vi "AlliGator Compute Multiple Average Phasors (Selected Plots).vi"(8 "error in (no error)":errorcluster, 9 "Phasor Frequency":dbl[unit]=160000000.0 format="%#_4g", 10 "Lifetime Graph Ref":refnum<vi>, 11 "Phasor Graph Ref":refnum<vi>) -> (0 "error out":errorcluster, 1 "Phasor SDV Plot":cluster{"Array":dbl[], "Array":dbl[]}, 2 "Average Phasor Plot":cluster{"Array":dbl[], "Array":dbl[]}, 4 "Result String":string)   [LabVIEW 2021, in "AlliGator Phasor Graph.lvlib"]
doc: "Computes one average phasor (and derived quantities) per phasor plot in the Phasor Graph and plots each quantity as a series (where the abscissa is the plot index)."
uses:
  AlliGator Phasor Graph.lvlib
  Phasor/Phasor (g, s).ctl
  71c37bd2-47c7-4488-96cd-0a664e0032d0.vi/bdeb4727-ff4d-4ac9-8e28-741831c2f97b.vi
  71c37bd2-47c7-4488-96cd-0a664e0032d0.vi/144b8a7a-6b33-495e-8c76-f9961f20cf57.vi
  71c37bd2-47c7-4488-96cd-0a664e0032d0.vi/b7572d45-ec39-4925-b449-50494e6a70fe.vi
  71c37bd2-47c7-4488-96cd-0a664e0032d0.vi/1eb0ddea-bb1c-44e5-a105-a57d15a7e766.vi
  71c37bd2-47c7-4488-96cd-0a664e0032d0.vi/c6722fb2-ba6a-4669-88ce-b6a529e82caa.vi
  71c37bd2-47c7-4488-96cd-0a664e0032d0.vi/9c66b583-3c03-4ab0-9ee8-bb1b5672edcc.vi
  71c37bd2-47c7-4488-96cd-0a664e0032d0.vi/fa4085e0-ed61-4e8f-9831-aca6a4188fed.vi
  71c37bd2-47c7-4488-96cd-0a664e0032d0.vi/0c4d34e2-59e2-4c6b-a2f9-6f475d8bea3b.vi
  71c37bd2-47c7-4488-96cd-0a664e0032d0.vi/9179bf7b-4f23-4b71-844f-7bfb33db4ee4.vi
  af37836b-9043-4320-9d11-d8691fee8c1a.vi/bdeb4727-ff4d-4ac9-8e28-741831c2f97b.vi
  af37836b-9043-4320-9d11-d8691fee8c1a.vi/144b8a7a-6b33-495e-8c76-f9961f20cf57.vi
  af37836b-9043-4320-9d11-d8691fee8c1a.vi/b7572d45-ec39-4925-b449-50494e6a70fe.vi
  af37836b-9043-4320-9d11-d8691fee8c1a.vi/1eb0ddea-bb1c-44e5-a105-a57d15a7e766.vi
  af37836b-9043-4320-9d11-d8691fee8c1a.vi/c6722fb2-ba6a-4669-88ce-b6a529e82caa.vi
  af37836b-9043-4320-9d11-d8691fee8c1a.vi/9c66b583-3c03-4ab0-9ee8-bb1b5672edcc.vi
  af37836b-9043-4320-9d11-d8691fee8c1a.vi/fa4085e0-ed61-4e8f-9831-aca6a4188fed.vi
  af37836b-9043-4320-9d11-d8691fee8c1a.vi/0c4d34e2-59e2-4c6b-a2f9-6f475d8bea3b.vi
  af37836b-9043-4320-9d11-d8691fee8c1a.vi/9179bf7b-4f23-4b71-844f-7bfb33db4ee4.vi
  bb80a456-60a4-403d-849e-61bda53aa3b6.vi/bdeb4727-ff4d-4ac9-8e28-741831c2f97b.vi
  bb80a456-60a4-403d-849e-61bda53aa3b6.vi/144b8a7a-6b33-495e-8c76-f9961f20cf57.vi
  bb80a456-60a4-403d-849e-61bda53aa3b6.vi/b7572d45-ec39-4925-b449-50494e6a70fe.vi
  bb80a456-60a4-403d-849e-61bda53aa3b6.vi/1eb0ddea-bb1c-44e5-a105-a57d15a7e766.vi
  bb80a456-60a4-403d-849e-61bda53aa3b6.vi/c6722fb2-ba6a-4669-88ce-b6a529e82caa.vi
  bb80a456-60a4-403d-849e-61bda53aa3b6.vi/9c66b583-3c03-4ab0-9ee8-bb1b5672edcc.vi
  bb80a456-60a4-403d-849e-61bda53aa3b6.vi/fa4085e0-ed61-4e8f-9831-aca6a4188fed.vi
  bb80a456-60a4-403d-849e-61bda53aa3b6.vi/0c4d34e2-59e2-4c6b-a2f9-6f475d8bea3b.vi
  bb80a456-60a4-403d-849e-61bda53aa3b6.vi/9179bf7b-4f23-4b71-844f-7bfb33db4ee4.vi
  4a9871b1-e52c-439f-b7fd-fdf7bfeb4803.vi/bdeb4727-ff4d-4ac9-8e28-741831c2f97b.vi
  4a9871b1-e52c-439f-b7fd-fdf7bfeb4803.vi/144b8a7a-6b33-495e-8c76-f9961f20cf57.vi
  4a9871b1-e52c-439f-b7fd-fdf7bfeb4803.vi/b7572d45-ec39-4925-b449-50494e6a70fe.vi
  4a9871b1-e52c-439f-b7fd-fdf7bfeb4803.vi/1eb0ddea-bb1c-44e5-a105-a57d15a7e766.vi
  4a9871b1-e52c-439f-b7fd-fdf7bfeb4803.vi/c6722fb2-ba6a-4669-88ce-b6a529e82caa.vi
  4a9871b1-e52c-439f-b7fd-fdf7bfeb4803.vi/9c66b583-3c03-4ab0-9ee8-bb1b5672edcc.vi
  4a9871b1-e52c-439f-b7fd-fdf7bfeb4803.vi/fa4085e0-ed61-4e8f-9831-aca6a4188fed.vi
  4a9871b1-e52c-439f-b7fd-fdf7bfeb4803.vi/0c4d34e2-59e2-4c6b-a2f9-6f475d8bea3b.vi
  4a9871b1-e52c-439f-b7fd-fdf7bfeb4803.vi/9179bf7b-4f23-4b71-844f-7bfb33db4ee4.vi
  ea11824e-7dc4-44cf-8e7c-2ee366fc47de.vi/bdeb4727-ff4d-4ac9-8e28-741831c2f97b.vi
  ea11824e-7dc4-44cf-8e7c-2ee366fc47de.vi/144b8a7a-6b33-495e-8c76-f9961f20cf57.vi
  ea11824e-7dc4-44cf-8e7c-2ee366fc47de.vi/b7572d45-ec39-4925-b449-50494e6a70fe.vi
  ea11824e-7dc4-44cf-8e7c-2ee366fc47de.vi/1eb0ddea-bb1c-44e5-a105-a57d15a7e766.vi
  ea11824e-7dc4-44cf-8e7c-2ee366fc47de.vi/c6722fb2-ba6a-4669-88ce-b6a529e82caa.vi
  ea11824e-7dc4-44cf-8e7c-2ee366fc47de.vi/9c66b583-3c03-4ab0-9ee8-bb1b5672edcc.vi
  ea11824e-7dc4-44cf-8e7c-2ee366fc47de.vi/fa4085e0-ed61-4e8f-9831-aca6a4188fed.vi
  ea11824e-7dc4-44cf-8e7c-2ee366fc47de.vi/0c4d34e2-59e2-4c6b-a2f9-6f475d8bea3b.vi
  ea11824e-7dc4-44cf-8e7c-2ee366fc47de.vi/9179bf7b-4f23-4b71-844f-7bfb33db4ee4.vi
  6682c489-6466-43b2-8f2f-8d331e8ea9c3.vi/bdeb4727-ff4d-4ac9-8e28-741831c2f97b.vi
  6682c489-6466-43b2-8f2f-8d331e8ea9c3.vi/144b8a7a-6b33-495e-8c76-f9961f20cf57.vi
  6682c489-6466-43b2-8f2f-8d331e8ea9c3.vi/b7572d45-ec39-4925-b449-50494e6a70fe.vi
  6682c489-6466-43b2-8f2f-8d331e8ea9c3.vi/1eb0ddea-bb1c-44e5-a105-a57d15a7e766.vi
  6682c489-6466-43b2-8f2f-8d331e8ea9c3.vi/c6722fb2-ba6a-4669-88ce-b6a529e82caa.vi
  6682c489-6466-43b2-8f2f-8d331e8ea9c3.vi/9c66b583-3c03-4ab0-9ee8-bb1b5672edcc.vi
  6682c489-6466-43b2-8f2f-8d331e8ea9c3.vi/fa4085e0-ed61-4e8f-9831-aca6a4188fed.vi
  6682c489-6466-43b2-8f2f-8d331e8ea9c3.vi/0c4d34e2-59e2-4c6b-a2f9-6f475d8bea3b.vi
  6682c489-6466-43b2-8f2f-8d331e8ea9c3.vi/9179bf7b-4f23-4b71-844f-7bfb33db4ee4.vi
  4c569add-43d7-45f2-8521-633ddc3d646c.vi/bdeb4727-ff4d-4ac9-8e28-741831c2f97b.vi
  4c569add-43d7-45f2-8521-633ddc3d646c.vi/144b8a7a-6b33-495e-8c76-f9961f20cf57.vi
  4c569add-43d7-45f2-8521-633ddc3d646c.vi/b7572d45-ec39-4925-b449-50494e6a70fe.vi
  4c569add-43d7-45f2-8521-633ddc3d646c.vi/1eb0ddea-bb1c-44e5-a105-a57d15a7e766.vi
  4c569add-43d7-45f2-8521-633ddc3d646c.vi/c6722fb2-ba6a-4669-88ce-b6a529e82caa.vi
  4c569add-43d7-45f2-8521-633ddc3d646c.vi/9c66b583-3c03-4ab0-9ee8-bb1b5672edcc.vi
  4c569add-43d7-45f2-8521-633ddc3d646c.vi/fa4085e0-ed61-4e8f-9831-aca6a4188fed.vi
  4c569add-43d7-45f2-8521-633ddc3d646c.vi/0c4d34e2-59e2-4c6b-a2f9-6f475d8bea3b.vi
  4c569add-43d7-45f2-8521-633ddc3d646c.vi/9179bf7b-4f23-4b71-844f-7bfb33db4ee4.vi
  2777646a-574b-4d4e-97c5-dbf227eafc7c.vi/bdeb4727-ff4d-4ac9-8e28-741831c2f97b.vi
  2777646a-574b-4d4e-97c5-dbf227eafc7c.vi/144b8a7a-6b33-495e-8c76-f9961f20cf57.vi
  2777646a-574b-4d4e-97c5-dbf227eafc7c.vi/b7572d45-ec39-4925-b449-50494e6a70fe.vi
  2777646a-574b-4d4e-97c5-dbf227eafc7c.vi/1eb0ddea-bb1c-44e5-a105-a57d15a7e766.vi
  2777646a-574b-4d4e-97c5-dbf227eafc7c.vi/c6722fb2-ba6a-4669-88ce-b6a529e82caa.vi
  2777646a-574b-4d4e-97c5-dbf227eafc7c.vi/9c66b583-3c03-4ab0-9ee8-bb1b5672edcc.vi
  2777646a-574b-4d4e-97c5-dbf227eafc7c.vi/fa4085e0-ed61-4e8f-9831-aca6a4188fed.vi
  2777646a-574b-4d4e-97c5-dbf227eafc7c.vi/0c4d34e2-59e2-4c6b-a2f9-6f475d8bea3b.vi
  2777646a-574b-4d4e-97c5-dbf227eafc7c.vi/9179bf7b-4f23-4b71-844f-7bfb33db4ee4.vi
  <userlib>/_OpenG.lib/array/array.llb/Filter 1D Array with Scalar (I32)__ogtk.vi
  AlliGator Abort.vi
  Graphs/XY Graph/XY Graph Add Single Plot with Name.vi
  <vilib>/Utility/error.llb/Error Cluster From Error Code.vi
  <vilib>/ErrorRing/Error Ring.xnode
  Phasor/Phasor.lvlib
  <vilib>/Analysis/NI_AALBase.lvlib
  Arrays/Arrays.lvlib
  Graphs/XY Graph/XY Graph Add-Ons.lvlib
  AlliGator Phasor Ratio.lvlib
  <userlib>/_OpenG.lib/array/array.llb/openg_array.lvlib
  AlliGator Globals, Variables & Constants.lvlib
  Strings/Strings.lvlib
  Utilities/Utilities.lvlib
  <userlib>/_OpenG.lib/array/array.llb/Filter 1D Array (DBL)__ogtk.vi
panel:
  # "see the AlliGator License on the block diagram (Ctrl+E or Window:Show Block Diagram)"
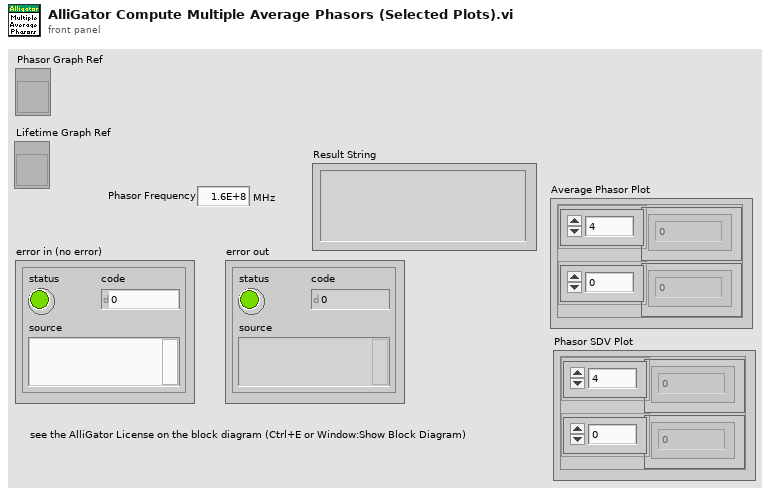
[diagram p1: front panel]
types:
  T1 = typedef "XY Graph Add-Ons.lvlib/XY Graph Refnum.ctl" = refnum<vi>
  T2 = typedef "Phasor.lvlib/Phasor (g, s).ctl" = cluster{"g":dbl, "s":dbl}
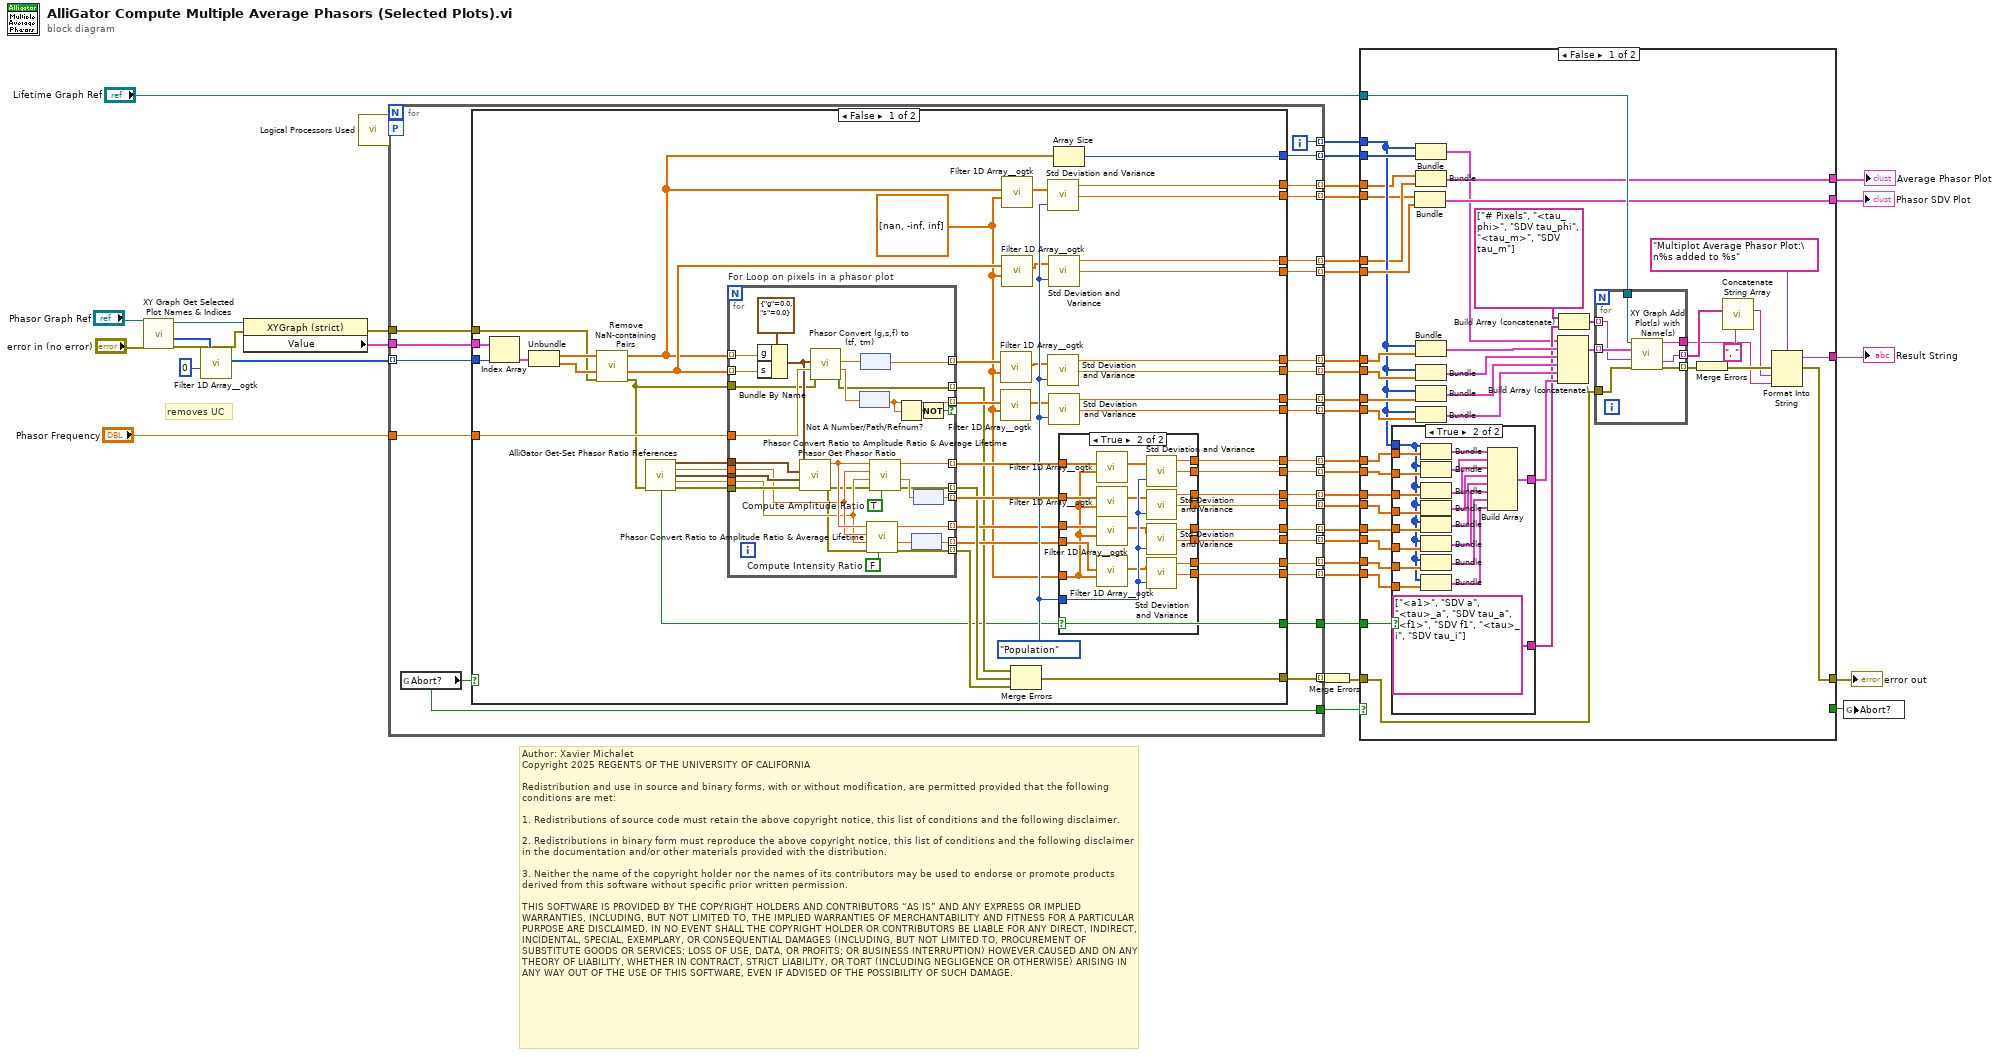
[diagram p0: block diagram]
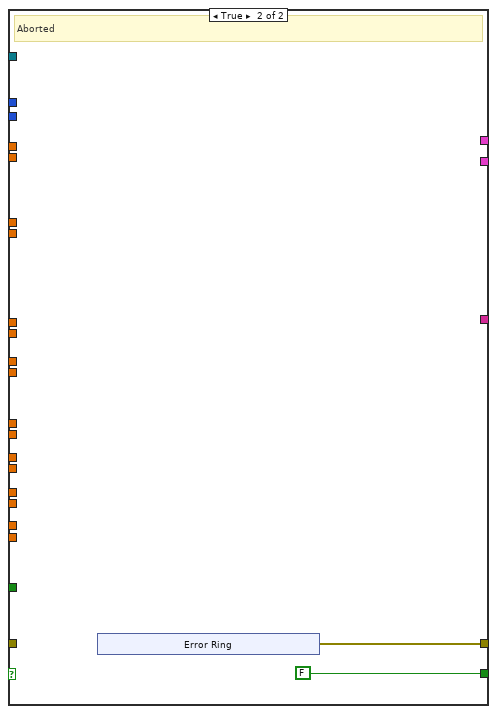
[diagram p3: hidden frame]
diagram:
  # "Author: Xavier Michalet\nCopyright 2025 REGENTS OF THE UNIVERSITY OF CALIFORNIA\n\nRedistribution and use in source and binary forms, with or without modification, are permitted provided that the following conditions are met:\n\n1. Redistributions of source code must retain the above copyright notice, this list of conditions and the following disclaimer.\n\n2. Redistributions in binary form must reproduce the above copyright notice, this list of conditions and the following disclaimer in the documentation and/or other materials provided with the distribution.\n\n3. Neither the name of the copyright holder nor the names of its contributors may be used to endorse or promote products derived from this software without specific prior written permission.\n\nTHIS SOFTWARE IS PROVIDED BY THE COPYRIGHT HOLDERS AND CONTRIBUTORS “AS IS” AND ANY EXPRESS OR IMPLIED WARRANTIES, INCLUDING, BUT NOT LIMITED TO, THE IMPLIED WARRANTIES OF MERCHANTABILITY AND FITNESS FOR A PARTICULAR PURPOSE ARE DISCLAIMED. IN NO EVENT SHALL THE COPYRIGHT HOLDER OR CONTRIBUTORS BE LIABLE FOR ANY DIRECT, INDIRECT, INCIDENTAL, SPECIAL, EXEMPLARY, OR CONSEQUENTIAL DAMAGES (INCLUDING, BUT NOT LIMITED TO, PROCUREMENT OF SUBSTITUTE GOODS OR SERVICES; LOSS OF USE, DATA, OR PROFITS; OR BUSINESS INTERRUPTION) HOWEVER CAUSED AND ON ANY THEORY OF LIABILITY, WHETHER IN CONTRACT, STRICT LIABILITY, OR TORT (INCLUDING NEGLIGENCE OR OTHERWISE) ARISING IN ANY WAY OUT OF THE USE OF THIS SOFTWARE, EVEN IF ADVISED OF THE POSSIBILITY OF SUCH DAMAGE."
  # "removes UC"
  n1 = call "XY Graph Get Selected Plot Names & Indices.vi"("error in (no error)"="error in (no error)", "XYGraph in"="Phasor Graph Ref") -> ("error out"=w5:errorcluster, "Selected Plots"=w36:i32[], "XYGraph out"=w6:T1)  [unwired: 5 in, 2 out]
  n2 = call-poly <userlib>:"Filter 1D Array__ogtk.vi"("items to filter"=0, "array"=w36) -> ("filtered array"=w34:i32[])  [unwired: 4 in, 1 out]
  n3 = property class="XYGraph (strict)"(reference=w6, error in=w5) -> (error out=w4:errorcluster, "Value"=w3:cluster{"X Array":dbl[], "Y Array":dbl[]}[])  [unwired: 1 out]
  n4 = call "Logical Processors Used.vi"() -> ("# Logical Processor Used"=w13:i32)  [unwired: 6 in]
  n5 = for {
    tunnel: "Phasor Frequency" -> [w64]
    tunnel: w4 -> [w63]
    tunnel: w34 -> [w62] mode=indexing
    tunnel: [w61] -> w33 mode=indexing
    tunnel: [w60] -> w31 mode=indexing
    tunnel: [w59] -> w30 mode=indexing
    tunnel: [w58] -> w29 mode=indexing
    tunnel: [w57] -> w28 mode=indexing
    tunnel: [w56] -> w27 mode=indexing
    tunnel: [w55] -> w26 mode=indexing
    tunnel: [w54] -> w25 mode=indexing
    tunnel: [w53] -> w24 mode=indexing
    tunnel: [w52] -> w23 mode=indexing
    tunnel: [w51] -> w22 mode=indexing
    tunnel: [w50] -> w21 mode=indexing
    tunnel: [w49] -> w20 mode=indexing
    tunnel: [w48] -> w19 mode=indexing
    tunnel: [w47] -> w18 mode=indexing
    tunnel: [w46] -> w17 mode=indexing
    tunnel: [w45] -> w32 mode=indexing
    tunnel: [w44] -> w16 mode=indexing
    tunnel: [w43] -> w10 mode=indexing
    tunnel: [w42] -> w15
    workers-P: w13 -> [_]
    tunnel: [w41] -> w12
    tunnel: w3 -> [w40]
    i -> [w44]
    n6 = global read "AlliGator Abort.vi" "Abort?"() -> (w41:bool)
    n7 = case shown="False" w41 {
      tunnel: w64 -> [w111 _]
      tunnel: w63 -> [w66 _]
      tunnel: w62 -> [w68 _]
      tunnel: [w87 _] -> w61
      tunnel: [w86 _] -> w60
      tunnel: [w85 _] -> w59
      tunnel: [w84 _] -> w58
      tunnel: [w83 _] -> w57
      tunnel: [w82 _] -> w56
      tunnel: [w81 _] -> w55
      tunnel: [w80 _] -> w54
      tunnel: [w79 _] -> w53
      tunnel: [w78 _] -> w52
      tunnel: [w77 _] -> w51
      tunnel: [w76 _] -> w50
      tunnel: [w75 _] -> w49
      tunnel: [w74 _] -> w48
      tunnel: [w73 _] -> w47
      tunnel: [w72 _] -> w46
      tunnel: [w70 _] -> w45
      tunnel: [w69 _] -> w43
      tunnel: [w65 _] -> w42
      tunnel: w40 -> [w67 _]
      frame False {
        w90 = dbl[] [nan, -inf, inf] ("Element(s) to Remove")
        w103 = enum16{"Sample", "Population"}."Population" ("Weighting (Sample)")
        n8 = Index Array(array=w67, index=w68) -> (element=w88:cluster{"X Array":dbl[], "Y Array":dbl[]})
        n9 = Unbundle(w88) -> ("X Array"=w113:dbl[], "Y Array"=w112:dbl[])
        n10 = call "Remove NaN-containing Pairs.vi"("Error In"=w66, "Y Array in"=w112, "X Array in"=w113) -> ("Error Out"=w91:errorcluster, "Y Array out"=w98:dbl[], "X Array out"=w71:dbl[])  [unwired: 5 in, 1 out]
        n11 = call "AlliGator Get-Set Phasor Ratio References.vi"("error in (no error)"=w91) -> ("All defined?"=w65:bool, "Reference Phasor 1"=w108:T2, "Reference Lifetime 1"=w106:dbl[unit], "Reference Phasor 2"=w107:T2, "Reference Lifetime 2"=w105:dbl[unit], "error out"=w110:errorcluster)  [unwired: 7 in, 2 out]
        n12 = for "For Loop on pixels in a phasor plot" {
          tunnel: w98 -> [w159] mode=indexing
          tunnel: w71 -> [w160] mode=indexing
          tunnel: w111 -> [w157]
          tunnel: [w158] -> w96 mode=indexing
          tunnel: [w154] -> w94 mode=indexing if=w152
          tunnel: w110 -> [w151]
          tunnel: w107 -> [w150]
          tunnel: w108 -> [w149]
          tunnel: w105 -> [w140]
          tunnel: w106 -> [w141]
          tunnel: [w147] -> w104 mode=indexing
          tunnel: [w144] -> w109 mode=indexing
          tunnel: [w145] -> w102 mode=indexing
          tunnel: [w137] -> w101 mode=indexing
          tunnel: [w135] -> w100 mode=indexing
          tunnel: [w134] -> w92 mode=indexing
          tunnel: w91 -> [w133]
          tunnel: [w132] -> w89 mode=indexing
          w138 = FALSE  # Compute Intensity Ratio
          w143 = TRUE  # Compute Amplitude Ratio
          n13 = Bundle By Name(cluster=T2 {"g"=0.0, "s"=0.0} ("Phasor (g, s)"), "g"=w160, "s"=w159) -> (w148:T2)
          n14 = call "Phasor Get Phasor Ratio.vi"("Error In"=w151, "Reference Phasor 2"=w150, "Reference Phasor 1"=w149, "Phasor"=w148) -> ("Error Out"=w139:errorcluster, "Phasor Ratio (f1)"=w142:dbl)  [unwired: 5 in, 1 out]
          n15 = call "Phasor Convert (g,s,f) to (tf, tm).vi"("Error In"=w133, "Phasor Harmonic Frequency"=w157, "Phasor (g, s)"=w148) -> ("Error Out"=w132:errorcluster, "Modulus Lifetime"=w155:dbl[unit], "Phase Lifetime"=w156:dbl[unit])  [unwired: 6 in]
          n16 = node(w155) -> (w154:dbl)
          n17 = node(w156) -> (w158:dbl)
          n18 = call "Phasor Convert Ratio to Amplitude Ratio & Average Lifetime.vi"("Compute Amplitude Ratio"=w138, "error in (no error)"=w139, "Reference Lifetime 2"=w140, "Reference Lifetime 1"=w141, "Phasor Ratio (f1)"=w142) -> ("error out"=w134:errorcluster, "Average Lifetime"=w136:dbl[unit], "Phasor/Amplitude Ratio"=w137:dbl)  [unwired: 2 in, 2 out]
          n19 = call "Phasor Convert Ratio to Amplitude Ratio & Average Lifetime.vi"("Compute Amplitude Ratio"=w143, "error in (no error)"=w139, "Reference Lifetime 2"=w140, "Reference Lifetime 1"=w141, "Phasor Ratio (f1)"=w142) -> ("error out"=w145:errorcluster, "Average Lifetime"=w146:dbl[unit], "Phasor/Amplitude Ratio"=w147:dbl)  [unwired: 2 in, 2 out]
          n20 = Not A Number/Path/Refnum?(number/path/refnum=w154) -> (NaN/Path/Refnum?=w153:bool)
          n21 = node(w136) -> (w135:dbl)
          n22 = node(w146) -> (w144:dbl)
          n23 = Not(x=w153) -> (.not. x?=w152:bool)
        }
        n24 = call-poly <userlib>:"Filter 1D Array__ogtk.vi"("items to filter"=w90, "array"=w94) -> ("filtered array"=w93:dbl[])  [unwired: 4 in, 1 out]
        n25 = call-poly <userlib>:"Filter 1D Array__ogtk.vi"("items to filter"=w90, "array"=w96) -> ("filtered array"=w95:dbl[])  [unwired: 4 in, 1 out]
        n26 = call-poly <userlib>:"Filter 1D Array__ogtk.vi"("items to filter"=w90, "array"=w71) -> ("filtered array"=w99:dbl[])  [unwired: 4 in, 1 out]
        n27 = call-poly <userlib>:"Filter 1D Array__ogtk.vi"("items to filter"=w90, "array"=w98) -> ("filtered array"=w97:dbl[])  [unwired: 4 in, 1 out]
        n28 = Merge Errors(w89, w102, w92) -> (w69:errorcluster)
        n29 = call <vilib>:"Std Deviation and Variance.vi"("X"=w99, "Weighting (Sample)"=w103) -> ("mean"=w87:dbl, "standard deviation"=w86:dbl)  [unwired: 1 out]
        n30 = call <vilib>:"Std Deviation and Variance.vi"("X"=w95, "Weighting (Sample)"=w103) -> ("mean"=w83:dbl, "standard deviation"=w82:dbl)  [unwired: 1 out]
        n31 = call <vilib>:"Std Deviation and Variance.vi"("X"=w97, "Weighting (Sample)"=w103) -> ("mean"=w85:dbl, "standard deviation"=w84:dbl)  [unwired: 1 out]
        n32 = call <vilib>:"Std Deviation and Variance.vi"("X"=w93, "Weighting (Sample)"=w103) -> ("mean"=w81:dbl, "standard deviation"=w80:dbl)  [unwired: 1 out]
        n33 = Array Size(array=w71) -> (size(s)=w70:i32)
        n34 = case shown="True" w65 {
          tunnel: w109 -> [_ w128]
          tunnel: w104 -> [_ w130]
          tunnel: w103 -> [_ w131]
          tunnel: w101 -> [_ w126]
          tunnel: w100 -> [_ w124]
          tunnel: w90 -> [_ w122]
          tunnel: [_ w121] -> w79
          tunnel: [_ w120] -> w78
          tunnel: [_ w119] -> w77
          tunnel: [_ w118] -> w76
          tunnel: [_ w117] -> w75
          tunnel: [_ w116] -> w74
          tunnel: [_ w115] -> w73
          tunnel: [_ w114] -> w72
          frame False {
          }
          frame True {
            n35 = call-poly <userlib>:"Filter 1D Array__ogtk.vi"("items to filter"=w122, "array"=w130) -> ("filtered array"=w129:dbl[])  [unwired: 4 in, 1 out]
            n36 = call-poly <userlib>:"Filter 1D Array__ogtk.vi"("items to filter"=w122, "array"=w128) -> ("filtered array"=w127:dbl[])  [unwired: 4 in, 1 out]
            n37 = call-poly <userlib>:"Filter 1D Array__ogtk.vi"("items to filter"=w122, "array"=w126) -> ("filtered array"=w125:dbl[])  [unwired: 4 in, 1 out]
            n38 = call-poly <userlib>:"Filter 1D Array__ogtk.vi"("items to filter"=w122, "array"=w124) -> ("filtered array"=w123:dbl[])  [unwired: 4 in, 1 out]
            n39 = call <vilib>:"Std Deviation and Variance.vi"("X"=w129, "Weighting (Sample)"=w131) -> ("mean"=w121:dbl, "standard deviation"=w120:dbl)  [unwired: 1 out]
            n40 = call <vilib>:"Std Deviation and Variance.vi"("X"=w127, "Weighting (Sample)"=w131) -> ("mean"=w119:dbl, "standard deviation"=w118:dbl)  [unwired: 1 out]
            n41 = call <vilib>:"Std Deviation and Variance.vi"("X"=w125, "Weighting (Sample)"=w131) -> ("mean"=w117:dbl, "standard deviation"=w116:dbl)  [unwired: 1 out]
            n42 = call <vilib>:"Std Deviation and Variance.vi"("X"=w123, "Weighting (Sample)"=w131) -> ("mean"=w115:dbl, "standard deviation"=w114:dbl)  [unwired: 1 out]
          }
        }
      }
      frame True {
        # "Aborted"
      }
    }
  }
  n43 = Merge Errors(w10) -> (w9:errorcluster)
  n44 = case shown="False" w12 {
    tunnel: w33 -> [w187 _]
    tunnel: w32 -> [w203 _]
    tunnel: w31 -> [w185 _]
    tunnel: w30 -> [w186 _]
    tunnel: w29 -> [w202 _]
    tunnel: w28 -> [w201 _]
    tunnel: w27 -> [w200 _]
    tunnel: w26 -> [w199 _]
    tunnel: w25 -> [w198 _]
    tunnel: w24 -> [w197 _]
    tunnel: w23 -> [w196 _]
    tunnel: w22 -> [w195 _]
    tunnel: w21 -> [w194 _]
    tunnel: w20 -> [w193 _]
    tunnel: w19 -> [w192 _]
    tunnel: w18 -> [w191 _]
    tunnel: w17 -> [w190 _]
    tunnel: w16 -> [w189 _]
    tunnel: w15 -> [w188 _]
    tunnel: "Lifetime Graph Ref" -> [w175 _]
    tunnel: [_ FALSE ("Abort?")] -> w11
    tunnel: w9 -> [w176 _]
    tunnel: [w172 w230] -> w8
    tunnel: [w165 _] -> w7
    tunnel: [w164 _] -> w2
    tunnel: [w163 _] -> w1
    frame False {
      n45 = case shown="True" w188 {
        tunnel: w197 -> [_ w229]
        tunnel: w196 -> [_ w228]
        tunnel: w195 -> [_ w227]
        tunnel: w194 -> [_ w226]
        tunnel: w193 -> [_ w225]
        tunnel: w192 -> [_ w224]
        tunnel: w191 -> [_ w223]
        tunnel: w190 -> [_ w222]
        tunnel: w189 -> [_ w221]
        tunnel: [_ w212] -> w179
        tunnel: [_ string[] ["<a1>", "SDV a", "<tau>_a", "SDV tau_a", "<f1>", "SDV f1", "<tau>_i", "SDV tau_i"]] -> w178
        frame False {
        }
        frame True {
          n46 = Bundle(w221, w229) -> (w220:cluster{i32[], dbl[]})  [unwired: 1 in]
          n47 = Bundle(w221, w228) -> (w219:cluster{i32[], dbl[]})  [unwired: 1 in]
          n48 = Bundle(w221, w227) -> (w218:cluster{i32[], dbl[]})  [unwired: 1 in]
          n49 = Bundle(w221, w226) -> (w217:cluster{i32[], dbl[]})  [unwired: 1 in]
          n50 = Bundle(w221, w225) -> (w216:cluster{i32[], dbl[]})  [unwired: 1 in]
          n51 = Bundle(w221, w224) -> (w215:cluster{i32[], dbl[]})  [unwired: 1 in]
          n52 = Bundle(w221, w223) -> (w214:cluster{i32[], dbl[]})  [unwired: 1 in]
          n53 = Bundle(w221, w222) -> (w213:cluster{i32[], dbl[]})  [unwired: 1 in]
          n54 = Build Array(w220, w219, w218, w217, w216, w215, w214, w213) -> (w212:cluster{i32[], dbl[]}[])
        }
      }
      n55 = Bundle(w185, w202) -> (w164:cluster{dbl[], dbl[]})  [unwired: 1 in]
      n56 = Bundle(w189, w203) -> (w162:cluster{i32[], i32[]})  [unwired: 1 in]
      n57 = Bundle(w187, w186) -> (w163:cluster{dbl[], dbl[]})  [unwired: 1 in]
      n58 = Bundle(w189, w201) -> (w184:cluster{i32[], dbl[]})  [unwired: 1 in]
      n59 = Bundle(w189, w200) -> (w182:cluster{i32[], dbl[]})  [unwired: 1 in]
      n60 = Bundle(w189, w199) -> (w181:cluster{i32[], dbl[]})  [unwired: 1 in]
      n61 = Bundle(w189, w198) -> (w180:cluster{i32[], dbl[]})  [unwired: 1 in]
      n62 = Build Array (concatenate)(w162, w184, w182, w181, w180, w179) -> (w183:cluster{i32[], dbl[]}[])
      n63 = Build Array (concatenate)(string[] ["# Pixels", "<tau_phi>", "SDV tau_phi", "<tau_m>", "SDV tau_m"], w178) -> (w177:string[])
      n64 = for {
        tunnel: w183 -> [w210] mode=indexing
        tunnel: w177 -> [w209] mode=indexing
        tunnel: w176 -> [w208]
        tunnel: w175 -> [w207]
        tunnel: [w206] -> w174 mode=indexing
        tunnel: [w205] -> w171 mode=indexing
        tunnel: [w204] -> w167
        n65 = call-poly "XY Graph Add Plot(s) with Name(s).vi"("XYGraph Ref in"=w207, "Plot"=w210, "Plot Name (\"Plot\")"=w209, "error in (no error)"=w208) -> ("XY Graph Caption (or Label)"=w204:string, "Plot Name"=w205:string, "error out"=w206:errorcluster)  [unwired: 8 in, 1 out]
      }
      n66 = Merge Errors(w174) -> (w173:errorcluster)
      n67 = call "Concatenate String Array.vi"("Separator (TAB)"=", ", "String Array"=w171) -> ("Formatted String"=w169:string)  [unwired: 9 in]
      n68 = Format Into String(format string="Multiplot Average Phasor Plot:\n%s added to %s", error in=w173, w169, w167) -> (resulting string=w165:string, error out=w172:errorcluster)  [unwired: 1 in]
    }
    frame True {
      # "Aborted"
      n69 = xnode "Error Ring"() -> ("error out"=w230:errorcluster)
    }
  }
  "error out" <- w8
  "Result String" <- w7
  "Average Phasor Plot" <- w1
  "Phasor SDV Plot" <- w2
  n70 = global write "AlliGator Abort.vi" "Abort?"(w11) -> ()
